vi "creat a file with first line.vi"(11 "file path (use dialog)":path) -> (0 "error out":errorcluster, 3 "Byte Stream File out":refnum<file>)   [LabVIEW 2015]
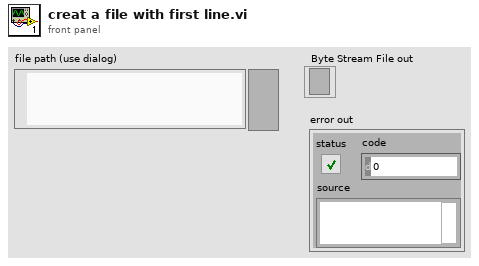
[diagram p1: front panel]
types:
  T1 = enum16{"open", "replace", "create", "open or create", "replace or create", "replace or create with confirmation"}
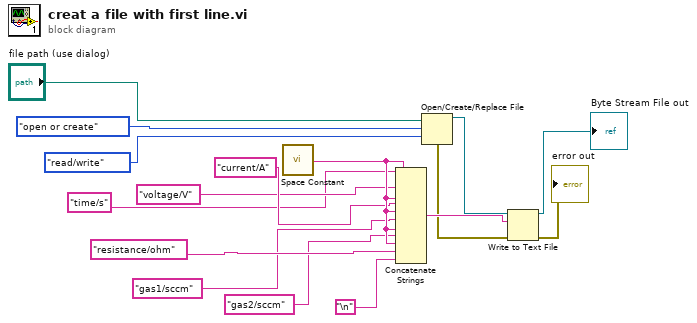
[diagram p0: block diagram]
diagram:
  n1 = call <vilib>:"Space Constant.vi"() -> ("String"=w15:string)
  n2 = Concatenate Strings("time/s" ("text"), w15, "voltage/V", w15, "current/A", w15, "gas1/sccm", w15, "gas2/sccm", w15, "resistance/ohm", "\n") -> (w11:string)
  n3 = Open/Create/Replace File(file path (use dialog)="file path (use dialog)", operation (0:open)=T1."open or create", access (0:read/write)=enum16{"read/write", "read-only", "write-only"}."read/write") -> (refnum out=w8:refnum<file>, error out=w10:errorcluster)  [unwired: 1 in, 3 out]
  n4 = Write to Text File(file (use dialog)=w8, text=w11, error in=w10) -> (refnum out=→"Byte Stream File out":refnum<file>, error out=→"error out":errorcluster)  [unwired: 1 in, 1 out]
